vi "Configure Modulation.vi"   [LabVIEW 2012, in "Novatech 409b.lvlib"]
doc: "Allows users to configure different modulation settings on the function generator."
uses:
  <instrlib>/Novatech 409b/Novatech 409b.lvlib
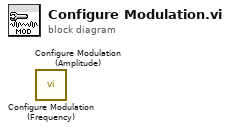
[diagram p0: block diagram]
diagram:
  n1 = call <instrlib>:"Configure Modulation (Frequency).vi"() -> ()  [unwired: 10 in, 2 out]
  n2 = call <instrlib>:"Configure Modulation (Amplitude).vi"() -> ()  [unwired: 10 in, 2 out]
